vi "fit_fix height and width.vi"() -> ()   [LabVIEW 2016] (continued)
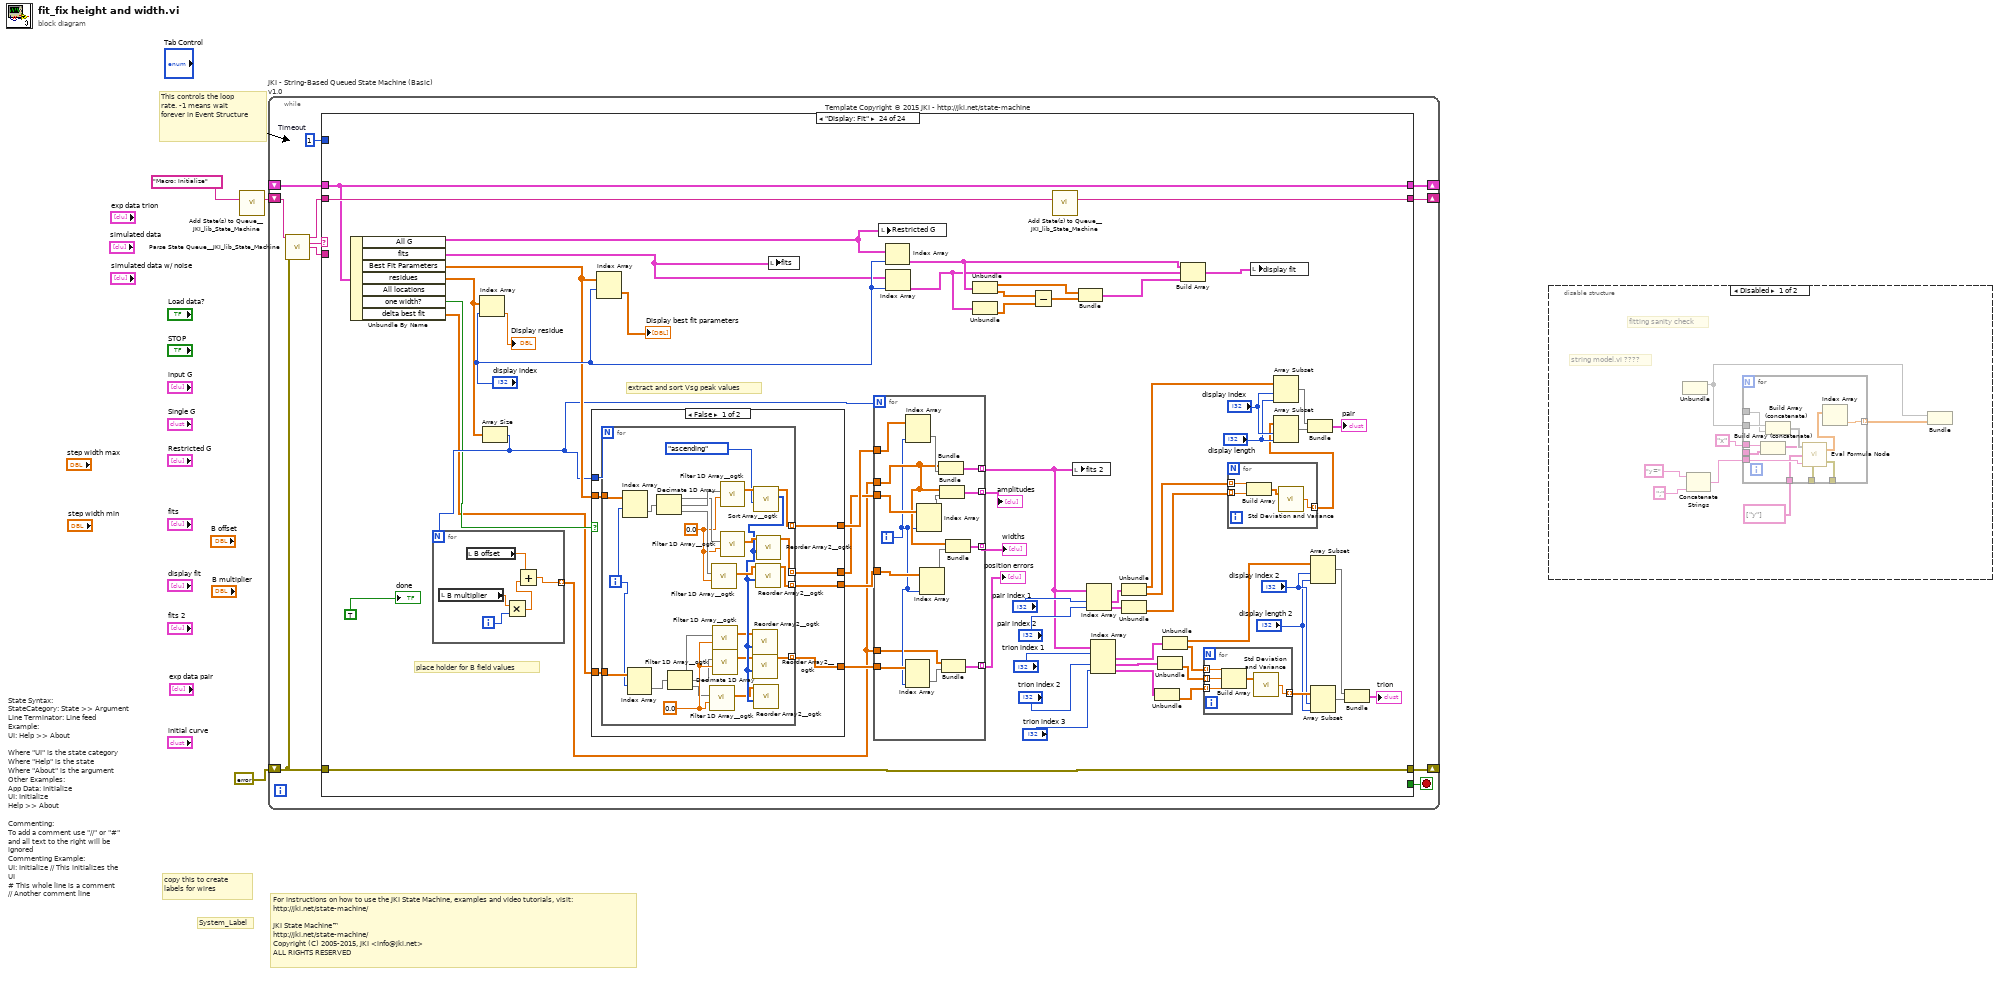
[diagram p0: block diagram]
diagram:
  # "For instructions on how to use the JKI State Machine, examples and video tutorials, visit:\nhttp://jki.net/state-machine/\n\nJKI State Machine™\nhttp://jki.net/state-machine/\nCopyright (C) 2005-2015, JKI <info@jki.net>\nALL RIGHTS RESERVED"
  # "State Syntax:\nStateCategory: State >> Argument\nLine Terminator: Line feed\nExample:\nUI: Help >> About\n\nWhere \"UI\" is the state category\nWhere \"Help\" is the state\nWhere \"About\" is the argument\nOther Examples:\nApp Data: Initialize\nUI: Initialize\nHelp >> About\n\nCommenting:\nTo add a comment use \"//\" or \"#\" and all text to the right will be ignored\nCommenting Example:\nUI: Initialize // This initializes the UI\n# This whole line is a comment\n// Another comment line"
  # "copy this to create labels for wires"
  # "This controls the loop rate. -1 means wait forever in Event Structure"
  # "System_Label"
  n1 = call <vilib>:"Add State(s) to Queue__JKI_lib_State_Machine.vi"("State(s) in (\"\")"="Macro: Initialize") -> ("States Out"=w3:string)  [unwired: 14 in]
  n2 = while "JKI - String-Based Queued State Machine (Basic) v1.0" {
    shift-right: [w7] -> _
    shift-left: _ -> [w6]
    shift-right: [w10] -> _
    shift-left: errorcluster {"status"=FALSE, "code"=0, "source"=""} ("error out") -> [w4]
    shift-right: [w9] -> _
    shift-left: w3 -> [w11]
    stop <- w8 stop-if-true
    w5 = 1  # Timeout
    # "Template Copyright © 2015 JKI - http://jki.net/state-machine"
    n3 = call <vilib>:"Parse State Queue__JKI_lib_State_Machine.vi"("State Queue"=w11, "Error In (no error)"=w4) -> ("Remaining States"=w13:string, "Current State"=w14:string, "Arguments"=w12:string)  [unwired: 11 in]
    n4 = case shown="\"Display: Fit\"" w14 {
      selector: w14 -> [_ _ w66 _ _ _ _ _ _ _ _ _ _ _ _ _ _ _ _ _ _ _ _ _]
      tunnel: w13 -> [w21 w65 w70 w88 w94 w100 w104 w135 w141 w145 w157 w163 w174 w200 w205 w215 w219 w248 w275 w312 w517 w593 w665 w726]
      tunnel: w12 -> [_ _ _ _ _ _ _ _ _ _ _ w158 w168 _ _ _ _ _ _ _ _ _ _ _]
      tunnel: w6 -> [w19 w62 w68 w79 w89 w98 w101 _ w136 w142 w154 w161 w170 w197 w202 w212 w216 w243 w271 w306 w511 w590 w662 w723]
      tunnel: [w18 w63 w72 w85 errorcluster {"status"=FALSE, "code"=0, "source"=""} ("error out") w97 w102 w132 w137 w143 w155 w159 w171 w198 w203 w213 w217 w246 w273 w310 w493 w589 w663 w720] -> w10
      tunnel: w4 -> [w17 w63 w71 w85 w90 w97 w102 w132 w138 w143 w155 w160 w172 w198 w203 w213 w217 w246 w273 w310 w510 w589 w663 w720]
      tunnel: [w20 w64 w69 w87 w93 w99 w103 w134 w140 w144 w156 w162 w173 w199 w204 w214 w218 w247 w274 w311 w516 w592 w664 w725] -> w9
      tunnel: [_ _ _ _ _ TRUE _ _ _ _ _ _ _ _ _ _ _ _ _ _ _ _ _ _] -> w8
      tunnel: [w16 w62 w68 w86 w89 w98 w101 w133 w136 w142 w152 w161 w170 w197 w202 w212 w216 w245 w270 w304 w514 w591 w662 w723] -> w7
      tunnel: w5 -> [w15 _ _ _ _ _ _ _ _ _ _ _ _ _ _ _ _ _ _ _ _ _ _ _]
      frame "", "Event Structure", "Idle" {
        # "executes when the state queue is empty"
        n5 = event shown="[0] Timeout" {
          selector: _ -> [_ _ _ _ _]
          dyn-events: _ -> [_ _ _ _ _]
          timeout: w15 -> [_ _ _ _ _]
          tunnel: w21 -> [w30 w35 w42 w55 w61]
          tunnel: [w29 w34 w41 w54 w60] -> w20
          tunnel: w19 -> [w24 w32 w38 w51 w58]
          tunnel: [w28 w33 w40 w53 w59] -> w18
          tunnel: w17 -> [w28 w33 w40 w53 w59]
          tunnel: [w22 w32 w39 w51 w58] -> w16
          event Timeout {
            n6 = event-data() -> ()  [unwired: 1 in, 1 out]
            n7 = local read "input G"() -> (w26:cluster{dbl[], dbl[]}[])
            n8 = Index Array(array=w26, index="choose initial curve") -> (element=w23:cluster{dbl[], dbl[]})
            n9 = Bundle By Name(cluster=w24, "initial curve"=w23) -> (w22:T5)
            n10 = local write "initial curve"(w23) -> ()
            n11 = call <vilib>:"Add State(s) to Queue__JKI_lib_State_Machine.vi"("State(s) in (\"\")"=w30, "State(s) at Back (\"\")"="Display: Fit" ("State(s) at Back (\"\")")) -> ("States Out"=w29:string)  [unwired: 13 in]
          }
          event "STOP": Value Change {
            # "Exit Button Value Change (pressed) Event\n(this executes Macro: Exit to terminate the VI)"
            n12 = event-data() -> ()  [unwired: 1 in, 1 out]
            n13 = call <vilib>:"Add State(s) to Queue__JKI_lib_State_Machine.vi"("State(s) in Front (\"\")"="Macro: Exit", "State(s) in (\"\")"=w35) -> ("States Out"=w34:string)  [unwired: 13 in]
          }
          event "Load data?": Value Change {
            n14 = event-data() -> ("NewVal"=w36:bool)  [unwired: 1 in, 5 out]
            n15 = case shown="True" w36 {
              tunnel: [w43 w50] -> w39
              tunnel: w38 -> [w43 w49]
              tunnel: [_ "UI: Initialize\nAnalysis: Load data"] -> w37
              frame False {
              }
              frame True {
                w47 = FALSE ("Done?")
                n16 = local write "done"(w47) -> ()
                n17 = Bundle By Name(cluster=w49, "curve #"=0, "Done?"=w47, "fits"=cluster{dbl[], dbl[]}[] [], "Initial curve?"=TRUE) -> (w50:T5)
              }
            }
            n18 = call <vilib>:"Add State(s) to Queue__JKI_lib_State_Machine.vi"("State(s) in Front (\"\")"=w37, "State(s) in (\"\")"=w42) -> ("States Out"=w41:string)  [unwired: 13 in]
          }
          event "display index": Value Change {
            n19 = event-data() -> ()  [unwired: 1 in, 6 out]
            n20 = call <vilib>:"Add State(s) to Queue__JKI_lib_State_Machine.vi"("State(s) in Front (\"\")"="Display: Fit", "State(s) in (\"\")"=w55) -> ("States Out"=w54:string)  [unwired: 13 in]
          }
          event Panel Close? {
            # "Discard the event because we'll close the front panel ourselves in Macro: Exit"
            # "Close Panel button (pressed) Event\n(this executes Macro: Exit to terminate the VI)"
            n21 = event-data() -> ()  [unwired: 1 in, 1 out]
            n22 = event-data("Discard?"=TRUE) -> ()  [unwired: 1 in, 1 out]
            n23 = call <vilib>:"Add State(s) to Queue__JKI_lib_State_Machine.vi"("State(s) in Front (\"\")"="Macro: Exit", "State(s) in (\"\")"=w61) -> ("States Out"=w60:string)  [unwired: 13 in]
          }
        }
      }
      frame "---------- Core ----------" {
        # "Do not put any code in this frame.\n(it is a separator no-op)"
        n24 = call <vilib>:"Add State(s) to Queue__JKI_lib_State_Machine.vi"("State(s) in (\"\")"=w65) -> ("States Out"=w64:string)  [unwired: 14 in]
      }
      frame Default {
        w75 = 42 items=["No error", "Argument error", "Memory is full", "Out of zone", "End of file", "File already open", "Generic file I/O error", "File not found", "File permission error", "Disk is full", "Duplicate path", "Too many files open", "System feature not enabled", "Resource file not found", "Cannot add resource", "Resource not found", "Image not found", "Image memory error", "Pen does not exist", "Config type invalid", "Config token not found", "Config parse error", "Config memory error", "Bad external code format", "Bad external code offset", "External code not present", "Null window", "Destroy window error", "Null menu", "Print aborted", "Bad print record", "Print driver error", "Windows error during printing", "Memory error during printing", "Print dialog error", "Generic print error", "Invalid device refnum", "Device not found", "Device parameter error", "Device unit error", "Cannot open device", "Device call aborted", "Generic error", "Cancelled by user", "Object ID too low", "Object ID too high", "Object not in heap", "Unknown heap", "Unknown object (invalid DefProc)", "Unknown object (DefProc not in table)", "Message out of range", "Invalid (null) method", "Unknown message", "Manager call not supported", "Bad address", "Network operation in progress", "Network operation timed out", "Connection is busy", "Network attribute not supported", "Network error", "Address in use", "System out of memory", "Connection aborted", "Connection refused", "Not connected", "Already connected", "Connection closed", "Initialization error (interapplication manager)", "Bad occurrence", "Wait on unbound occurrence handler", "Occurrence queue overflow", "Datalog type conflict", "Unused", "Unrecognized type (interapplication manager)", "Memory corrupt", "Failed to make temporary DLL", "Old CIN version", "Drag socket not found", "Failed to load drop-object", "Failed to register OLE object", "Failed to release OLE object", "Format specifier type mismatch", "Unknown format specifier", "Too few format specifiers", "Too many format specifiers", "Scan failed", "Newer CIN version", "Error converting to variant", "Runtime menu error", "Password tampered", "Variant attribute not found", "Incompatible variant data type", "Event data is not available", "Event Store is not present", "Occurrence is not found", "Event Queue is not created", "Event info is not available", "Refnum passed is NULL", "Error retrieving Class GUID", "Error retrieving CoClass GUID", "Error retrieving TypeLib GUID.", "Bad built application magic bytes.", "Specific driver is different from the specific driver associated with the Logical Name.", "There is no session opened to the class driver.", "Max Error", "MAX - Error with config objects", "MAX - Error loading configuration", "MAX - Group not supported"]
        # "Current State"
        # "Do not delete, rename, or modify this frame.\n(this is used to capture unhandled states and typos)"
        # "Handle mistyped state name (developer tool)"
        n25 = Format Into String(format string="Software Exception: Unhandled State \"%s\"." ("message"), error in=w71, w66) -> (resulting string=w74:string, error out=w73:errorcluster)  [unwired: 1 in]
        n26 = call <vilib>:"Error Cluster From Error Code.vi"("show call chain? (False)"=TRUE, "error in (no error)"=w73, "error message (\"\")"=w74, "error code (0)"=w75) -> ("error out"=w72:errorcluster)  [unwired: 5 in]
        n27 = call <vilib>:"Add State(s) to Queue__JKI_lib_State_Machine.vi"("State(s) in (\"\")"=w70) -> ("States Out"=w69:string)  [unwired: 14 in]
      }
      frame "Initialize Core Data" {
        # "Do not delete, rename, or modify this frame.\n(this is used to determine panel behavior on exit)"
        # "originally closed?"
        # "exe?"
        # "If panel starts closed or is an EXE, then close it when we exit"
        n28 = property class="App"() -> ("App.Kind"=w83:T3)  [unwired: 2 in, 2 out]
        n29 = property class="VI"() -> ("Front Panel.Open"=w84:bool)  [unwired: 2 in, 2 out]
        n30 = control-ref of="Current VI Reference"() -> (w77:refnum<vi>)
        n31 = Not(x=w84) -> (.not. x?=w81:bool)
        n32 = Equal?(x=w83, y=T3."Run Time System" ("Application:Kind")) -> (x = y?=w80:bool)
        n33 = Or(x=w81, y=w80) -> (x .or. y?=w78:bool)
        n34 = Bundle By Name(cluster=w79, "Core.Current VI Reference"=w77, "Core.Close Panel on Exit?"=w78) -> (w86:T5)
        n35 = call <vilib>:"Add State(s) to Queue__JKI_lib_State_Machine.vi"("State(s) in (\"\")"=w88) -> ("States Out"=w87:string)  [unwired: 14 in]
      }
      frame "Error Handler" {
        # "Unhandled Error -- Display it"
        # "Handle any errors here.\nYou can also output any states to clean-up after errors occur"
        # "Clear error"
        n36 = disable-structure shown="Disabled" {
          disable-tunnel: w90 -> [w95 _]
          frame Disabled {
            n37 = call <vilib>:"General Error Handler.vi"("error in (no error)"=w95) -> ()  [unwired: 10 in, 5 out]
          }
          frame Enabled {
          }
        }
        n38 = call <vilib>:"Add State(s) to Queue__JKI_lib_State_Machine.vi"("State(s) in (\"\")"=w94, "State(s) at Back (\"\")"="/* Post Error States") -> ("States Out"=w93:string)  [unwired: 13 in]
      }
      frame "Exit" {
        # "Do not put any code in this frame.\n(No errors that occur here will be handled.)"
        n39 = call <vilib>:"Add State(s) to Queue__JKI_lib_State_Machine.vi"("State(s) in (\"\")"=w100) -> ("States Out"=w99:string)  [unwired: 14 in]
      }
      frame "---------- Data ----------" {
        # "Do not put any code in this frame.\n(It is a separator no-op. You can make a copy of this frame to create a new Data frame)"
        n40 = call <vilib>:"Add State(s) to Queue__JKI_lib_State_Machine.vi"("State(s) in (\"\")"=w104) -> ("States Out"=w103:string)  [unwired: 14 in]
      }
      frame "Data: Initialize" {
        w105 = dbl[][] []  # delta best fit
        w106 = dbl[][] []  # Intermediate delta
        w107 = FALSE  # one width?
        w108 = i32[] []  # Fit steps
        w109 = dbl[][] []  # All locations
        w110 = dbl[] []  # Initial Best Fit
        w111 = FALSE  # Initial curve?
        w112 = cluster{"Single G curve":dbl[], dbl[]} {"Single G curve"=[], []}  # initial curve
        w114 = dbl[] []  # intermediate residues
        w115 = cluster{dbl[], dbl[]}[] []  # intermediate fits
        w116 = dbl[][] []  # Intermediate Best Fit
        w118 = 0  # fit iteration
        w119 = dbl[] []  # residues
        w120 = cluster{"max iteration":i32, "tolerance":dbl} {"max iteration"=200, "tolerance"=1e-08}  # termination
        w121 = T6 {"parameter minimum"=[], "parameter maximum"=[]}  # parameter bounds
        w122 = 0  # model step #
        w123 = dbl[][] []  # Best Fit Parameters
        w124 = dbl[] []  # Initial Parameters
        w125 = dbl[] []  # Locations
        w126 = dbl[] []  # Locations index
        w117 = -1  # curve #
        w127 = cluster{"Single G curve":dbl[], dbl[]} {"Single G curve"=[], []}  # Single G curve
        w128 = cluster{dbl[], dbl[]}[] []  # All G
        w129 = T7 {"Current VI Reference"=refnum, "Close Panel on Exit?"=FALSE}  # Core
        w131 = TRUE  # Done?
        w130 = ""  # Your string data
        # "Initialize the shift-register data, here.\n(data names are defined by what you wire into the bundle function)"
        n41 = local read "fits"() -> (w113:cluster{dbl[], dbl[]}[])
        n42 = call <vilib>:"Add State(s) to Queue__JKI_lib_State_Machine.vi"("State(s) in (\"\")"=w135) -> ("States Out"=w134:string)  [unwired: 14 in]
        n43 = Bundle("Core"=w129, "Done?"=w131, "Your string data"=w130, "All G"=w128, "Single G curve"=w127, "Locations index"=w126, "Locations"=w125, "Initial Parameters"=w124, "Best Fit Parameters"=w123, "Intermediate Best Fit"=w116, "curve #"=w117, "fits"=w113, "intermediate fits"=w115, "model step #"=w122, "parameter bounds"=w121, "termination"=w120, "residues"=w119, "intermediate residues"=w114, "fit iteration"=w118, "initial curve"=w112, "Initial curve?"=w111, "Initial Best Fit"=w110, "All locations"=w109, "Fit steps"=w108, "one width?"=w107, "delta best fit"=w105, "Intermediate delta"=w106) -> (w133:T5)  [unwired: 1 in]
      }
      frame "Data: Cleanup" {
        # "Cleanup any data and references, here.\n(this is called automatically, by the Macro: Exit)"
        n44 = Unbundle By Name(w136) -> ("Core.Current VI Reference"=w139:refnum<vi>)
        n45 = Close Reference(reference=w139, error in (no error)=w138) -> (error out=w137:errorcluster)
        n46 = call <vilib>:"Add State(s) to Queue__JKI_lib_State_Machine.vi"("State(s) in (\"\")"=w141) -> ("States Out"=w140:string)  [unwired: 14 in]
      }
      frame "---------- UI ----------" {
        # "Do not put any code in this frame.\n(It is a separator no-op. You can make a copy of this frame to create a new UI frame)"
        n47 = call <vilib>:"Add State(s) to Queue__JKI_lib_State_Machine.vi"("State(s) in (\"\")"=w145) -> ("States Out"=w144:string)  [unwired: 14 in]
      }
      frame "UI: Initialize" {
        # "default termination conditions"
        # "Initialize the User Interface, here.\n(this is called automatically, by the Macro: Init)"
        n48 = Bundle By Name(cluster=w154, "intermediate fits"=cluster{dbl[], dbl[]}[] [] ("fits"), "Best Fit Parameters"=dbl[][] [], "Intermediate Best Fit"=dbl[][] [] ("Best Fit Parameters"), "residues"=dbl[] [], "fit iteration"=0, "termination"=cluster{"max iteration":i32, "tolerance":dbl} {"max iteration"=200, "tolerance"=1e-08}, "Fit steps"=i32[] []) -> (w152:T5)
        n49 = call <vilib>:"Add State(s) to Queue__JKI_lib_State_Machine.vi"("State(s) in (\"\")"=w157) -> ("States Out"=w156:string)  [unwired: 14 in]
      }
      frame "UI: Cursor Set" {
        # "Argument"
        # "Set and Unset Cursor Busy.\n(Usage: \"UI: Cursor Set >> Busy|Idle\")"
        n50 = case shown="\"Idle\", Default" w158 {
          tunnel: w160 -> [w165 w167]
          tunnel: [w164 w166] -> w159
          frame "Idle", Default {
            n51 = call <vilib>:"Unset Busy.vi"("error in (no error)"=w165) -> ("error out"=w164:errorcluster)  [unwired: 10 in]
          }
          frame "Busy" {
            n52 = call <vilib>:"Set Busy.vi"("error in (no error)"=w167) -> ("error out"=w166:errorcluster)  [unwired: 9 in, 1 out]
          }
        }
        n53 = call <vilib>:"Add State(s) to Queue__JKI_lib_State_Machine.vi"("State(s) in (\"\")"=w163) -> ("States Out"=w162:string)  [unwired: 14 in]
      }
      frame "UI: Front Panel State" {
        # "Argument"
        # "Set Front Panel Open or Closed\n(Usage: \"UI: Front Panel State >> Open|Close\")"
        n54 = Unbundle By Name(w170) -> ("Core.Current VI Reference"=w169:refnum<vi>)
        n55 = case shown="\"Open\", Default" w168 {
          tunnel: w172 -> [w178 w191]
          tunnel: [w180 w192] -> w171
          tunnel: w169 -> [w179 w189]
          frame "Open", Default {
            n56 = property class="VI"(reference=w179, error in=w178) -> (reference out=w176:refnum<vi>, error out=w177:errorcluster, "Front Panel.Open"=w175:bool)
            n57 = case shown="False" w175 {
              tunnel: [w183 w186] -> w180
              tunnel: w177 -> [w182 w186]
              tunnel: w176 -> [w181 _]
              frame False {
                n58 = invoke class="VI" method="FP.Open"(reference=w181, error in=w182, "Activate"=TRUE, "State"=T4."Standard") -> (error out=w183:errorcluster)  [unwired: 1 in, 4 out]
              }
              frame True {
              }
            }
          }
          frame "Close" {
            n59 = property class="VI"(reference=w189, error in=w191) -> (reference out=w188:refnum<vi>, error out=w190:errorcluster, "Front Panel.Open"=w187:bool)
            n60 = case shown="True" w187 {
              tunnel: [w193 w196] -> w192
              tunnel: w190 -> [w193 w195]
              tunnel: w188 -> [_ w194]
              frame False {
              }
              frame True {
                n61 = invoke class="VI" method="FP.Close"(reference=w194, error in=w195) -> (error out=w196:errorcluster)  [unwired: 1 in, 2 out]
              }
            }
          }
        }
        n62 = call <vilib>:"Add State(s) to Queue__JKI_lib_State_Machine.vi"("State(s) in (\"\")"=w174) -> ("States Out"=w173:string)  [unwired: 14 in]
      }
      frame "---------- Macro ----------" {
        # "Do not put any code in this frame.\n(It is a separator no-op. You can make a copy of this frame to create a new Macro frame)"
        n63 = call <vilib>:"Add State(s) to Queue__JKI_lib_State_Machine.vi"("State(s) in (\"\")"=w200) -> ("States Out"=w199:string)  [unwired: 14 in]
      }
      frame "Macro: Initialize" {
        w201 = "Data: Initialize\nInitialize Core Data\nUI: Initialize\nUI: Front Panel State >> Open"  # Data: Initialize Initialize Core Data UI: Initialize UI: Front Panel State >> Open
        # "Initialization Macro\n(This is called once, when the VI starts)"
        n64 = call <vilib>:"Add State(s) to Queue__JKI_lib_State_Machine.vi"("State(s) in Front (\"\")"=w201, "State(s) in (\"\")"=w205) -> ("States Out"=w204:string)  [unwired: 13 in]
      }
      frame "Macro: Exit" {
        # "Exit Macro\n(This is called once, when the VI exits)"
        n65 = Unbundle By Name(w212) -> ("Core.Close Panel on Exit?"=w211:bool)
        n66 = Select(t="UI: Front Panel State >> Close", s=w211, f="") -> (s? t:f=w208:string)
        n67 = call <vilib>:"Add State(s) to Queue__JKI_lib_State_Machine.vi"("State(s) in (\"\")"=w208, "State(s) at Back (\"\")"="Data: Cleanup\nExit") -> ("States Out"=w206:string)  [unwired: 13 in]
        n68 = call <vilib>:"Add State(s) to Queue__JKI_lib_State_Machine.vi"("State(s) in Front (\"\")"=w206, "State(s) in (\"\")"=w215) -> ("States Out"=w214:string)  [unwired: 13 in]
      }
      frame "---------- Analysis ----------" {
        # "Template Separator\n(You can make a copy of, or modify, this frame)"
        n69 = call <vilib>:"Add State(s) to Queue__JKI_lib_State_Machine.vi"("State(s) in (\"\")"=w219) -> ("States Out"=w218:string)  [unwired: 14 in]
      }
      frame "Analysis: Load data" {
        # "Load data and step through curves for fitting"
        n70 = local read "input G"() -> (w230:cluster{dbl[], dbl[]}[])
        n71 = Unbundle By Name(w243) -> ("curve #"=w229:i32, "fit iteration"=w225:i32, "Initial curve?"=w233:bool)
        "curve #" <- w229
        n72 = Array Size(array=w230) -> (size(s)=w228:i32)
        n73 = Decrement(x=w228) -> (x-1=w227:i32)
        n74 = case shown="True" "Restrict G?" {
          tunnel: w230 -> [w249 w251]
          tunnel: [w249 w250] -> w242
          frame False {
          }
          frame True {
            n75 = for {
              tunnel: w251 -> [w259] mode=indexing
              tunnel: [w252] -> w250 mode=indexing
              n76 = Unbundle(w259) -> (w257:dbl[], w256:dbl[])
              n77 = Threshold 1D Array(2:"Max G", 3:w256) -> (0:w255:dbl)  [unwired: 1 in]
              n78 = Array Subset(array=w256, length=w255) -> (w253:dbl[])  [unwired: 1 in]
              n79 = Array Subset(array=w257, length=w255) -> (w254:dbl[])  [unwired: 1 in]
              n80 = Bundle(w254, w253) -> (w252:cluster{dbl[], dbl[]})  [unwired: 1 in]
            }
          }
        }
        n81 = Equal?(x=w229, y=w227) -> (x = y?=w226:bool)
        n82 = Equal?(x=w225, y=0) -> (x = y?=w223:bool)
        n83 = And(x=w226, y=w223) -> (x .and. y?=w222:bool)
        n84 = local read "choose initial curve"() -> (w232:i32)
        n85 = case shown="True" w222 {
          frame False {
          }
          frame True {
            n86 = call <vilib>:"Beep.vi"() -> ()  [unwired: 12 in]
          }
        }
        n87 = Select(t=w232, s=w233, f=w229) -> (s? t:f=w231:i32)
        n88 = Index Array(array=w242, index=w231) -> (element=w234:cluster{dbl[], dbl[]})
        n89 = local write "Single G"(w234) -> ()
        n90 = local write "Restricted G"(w242) -> ()
        n91 = Unbundle(w234) -> (w240:dbl[])  [unwired: 1 out]
        n92 = Array Max & Min(array=w240) -> (max value=w241:dbl)  [unwired: 3 out]
        n93 = Round Toward -Infinity(1:w241) -> (0:w221:dbl)
        n94 = Add(x=w221, y=w225) -> (x+y=w239:dbl)
        n95 = Bundle By Name(cluster=w243, "All G"=w242, "Single G curve"=w234, "model step #"=w239) -> (w245:T5)
        n96 = Equal?(x=0, y=w225) -> (x = y?=w237:bool)
        n97 = Select(t="Analysis: find peaks" ("State(s) at Back (\"\")"), s=w237, f="Analysis: Initial Parameters" ("State(s) at Back (\"\")")) -> (s? t:f=w220:string)
        n98 = call <vilib>:"Add State(s) to Queue__JKI_lib_State_Machine.vi"("State(s) in Front (\"\")"=w220, "State(s) in (\"\")"=w248) -> ("States Out"=w247:string)  [unwired: 13 in]
      }
      frame "Analysis: find peaks" {
        # "Fid peak locations to help constrain step position inital parameters"
        n99 = Unbundle By Name(w271) -> ("Single G curve"=w272:cluster{"Single G curve":dbl[], dbl[]})
        n100 = call <userlib>:"differential.vi"("Numeric"="derivative \nfor peak initial conditions", "dy/dx vs x"=TRUE, "A vs B 2"=w272) -> ("A vs B 3"=w267:T8)  [unwired: 1 in]
        n101 = Unbundle(w267) -> ("Decimated Array"=w263:dbl[], "Decimated Array"=w266:dbl[])
        n102 = call <vilib>:"Peak Detector.vi"("width"="derivative peak width", "threshold"="derivative peak threshold", "X"=w266) -> ("Locations"=w262:dbl[])  [unwired: 4 in, 4 out]
        "Locations index" <- w262
        n103 = for {
          N -> [w276]
          tunnel: w263 -> [w279]
          tunnel: w262 -> [w278] mode=indexing
          tunnel: [w277] -> w261 mode=indexing
          tunnel: [w276] -> _ mode=indexing
          n104 = Interpolate 1D Array(1:w278, 2:w279) -> (0:w277:dbl)
        }
        "Locations" <- w261
        n105 = call <vilib>:"Add State(s) to Queue__JKI_lib_State_Machine.vi"("State(s) in Front (\"\")"="Analysis: Initial Parameters" ("State(s) at Back (\"\")"), "State(s) in (\"\")"=w275) -> ("States Out"=w274:string)  [unwired: 13 in]
        n106 = Bundle By Name(cluster=w271, "Locations index"=w262, "Locations"=w261) -> (w270:T5)
      }
      frame "Analysis: Initial Parameters" {
        # "Create initial parameter and parameter bound arrays"
        n107 = Unbundle By Name(w306) -> ("Initial Best Fit"=w297:dbl[], "Initial curve?"=w288:bool, "model step #"=w301:i32, "Single G curve"=w309:cluster{"Single G curve":dbl[], dbl[]}, "Locations index"=w308:dbl[], "Locations"=w307:dbl[], "Best Fit Parameters"=w292:dbl[][], "residues"=w291:dbl[], "curve #"=w281:i32)
        n108 = case shown="True" "fix step width?" {
          tunnel: [w315 w316] -> w296
          tunnel: [w314 w316] -> w295
          tunnel: ["step width?" w316] -> w284
          tunnel: w281 -> [_ w324]
          frame False {
            n109 = local read "step width max"() -> (w315:dbl)
            n110 = local read "step width min"() -> (w314:dbl)
          }
          frame True {
            n111 = local read "B multiplier"() -> (w323:dbl)
            n112 = local read "B offset"() -> (w321:dbl)
            n113 = Multiply(x=w324, y=w323) -> (x*y=w322:dbl)
            n114 = Add(x=w322, y=w321) -> (x+y=w319:dbl)
            n115 = Multiply(x=w319, y="fix width slope") -> (x*y=w317:dbl)
            n116 = Add(x=w317, y="fix width intercept") -> (x+y=w316:dbl)
          }
        }
        n117 = Array Size(array=w291) -> (size(s)=w290:i32)
        n118 = Unbundle(w309) -> ("Single G curve"=w302:dbl[], w303:dbl[])
        n119 = Select(t=w288, s="fit inital parameters?", f=TRUE) -> (s? t:f=w287:bool)
        n120 = Decrement(x=w290) -> (x-1=w289:i32)
        n121 = case shown="True" w287 {
          tunnel: w308 -> [w339 w400]
          tunnel: w307 -> [w338 w399]
          tunnel: [w347 w398] -> w305
          tunnel: w303 -> [w341 w397]
          tunnel: w302 -> [w344 w396]
          tunnel: w301 -> [w351 w395]
          tunnel: [w337 w394] -> w300
          tunnel: [w345 w393] -> w299
          tunnel: w297 -> [w348 _]
          tunnel: w296 -> [w336 w392]
          tunnel: w295 -> [w335 w391]
          tunnel: "step height max" -> [w334 w390]
          tunnel: "step height min" -> [w333 w389]
          tunnel: w292 -> [w332 _]
          tunnel: w289 -> [w331 _]
          tunnel: "one width?" -> [_ w388]
          tunnel: w284 -> [_ w387]
          frame False {
            w346 = dbl[] []
            n122 = Index Array(array=w332, index (row)=w331) -> (element=w330:dbl[])  [unwired: 1 in]
            n123 = Array Max & Min(array=w344) -> (max value=w343:dbl, min value=w342:dbl)  [unwired: 2 out]
            n124 = call-poly <userlib>:"Filter 1D Array__ogtk.vi"("items to filter"=0.0, "array"=w348) -> ("filtered array"=w352:dbl[])  [unwired: 4 in, 1 out]
            n125 = Decimate 1D Array(w330) -> (w328:dbl[])  [unwired: 2 out]
            n126 = Multiply(x=w328, y="Max position %") -> (x*y=w326:dbl[])
            n127 = Multiply(x=w328, y="Min position %") -> (x*y=w325:dbl[])
            n128 = Decimate 1D Array(w352) -> (w350:dbl[], w349:dbl[])  [unwired: 1 out]
            n129 = for {
              N: w351 -> [_]
              tunnel: w350 -> [w386]
              tunnel: w349 -> [w385]
              shift-right: [w383] -> w347
              shift-left: dbl[] [] -> [w384]
              shift-right: [w381] -> w345
              shift-left: w346 -> [w382]
              shift-right: [w379] -> w337
              shift-left: w346 -> [w380]
              tunnel: w343 -> [w371]
              tunnel: w342 -> [w368]
              tunnel: w341 -> [w378]
              tunnel: w339 -> [w377]
              tunnel: w338 -> [w375]
              tunnel: w336 -> [w360]
              tunnel: w335 -> [w359]
              tunnel: w334 -> [w362]
              tunnel: w333 -> [w361]
              tunnel: w326 -> [w367]
              tunnel: w325 -> [w365]
              i -> [w364]
              n130 = Index Array(array=w367, index=w364) -> (element=w366:dbl)
              n131 = Index Array(array=w365, index=w364) -> (element=w363:dbl)
              n132 = Index Array(array=w386, index=w364) -> (element=w356:dbl)
              n133 = Index Array(array=w385, index=w364) -> (element=w372:dbl)
              n134 = Threshold 1D Array(2:w364, 3:w378) -> (0:w376:dbl)  [unwired: 1 in]
              n135 = call "compare if zero.vi"("if zero out"=w368, "Numeric"=w363) -> ("out"=w369:dbl)  [unwired: 5 in]
              n136 = call "compare if zero.vi"("if zero out"=w362, "Numeric"=w356) -> ("out"=w358:dbl)  [unwired: 5 in]
              n137 = call "compare if zero.vi"("if zero out"=w371, "Numeric"=w366) -> ("out"=w370:dbl)  [unwired: 5 in]
              n138 = call "Search 1D Array for Nearest LV2012 NIVerified.vi"("desired element"=w376, "1D Array"=w377) -> ("closest index"=w374:i32)  [unwired: 8 in, 1 out]
              n139 = call "compare if zero.vi"("if zero out"=w360, "Numeric"=w372) -> ("out"=w355:dbl)  [unwired: 5 in]
              n140 = call "compare if zero.vi"("if zero out"=w361, "Numeric"=w356) -> ("out"=w357:dbl)  [unwired: 5 in]
              n141 = call "compare if zero.vi"("if zero out"=w359, "Numeric"=w372) -> ("out"=w354:dbl)  [unwired: 5 in]
              n142 = Index Array(array=w375, index=w374) -> (element=w373:dbl)
              n143 = Build Array (concatenate)(w382, w358, w370, w355) -> (w381:dbl[])
              n144 = Build Array (concatenate)(w380, w357, w369, w354) -> (w379:dbl[])
              n145 = Build Array (concatenate)(w384, w356, w373, w372) -> (w383:dbl[])
            }
          }
          frame True {
            n146 = case shown="True" w388 {
              tunnel: w400 -> [w418 w453]
              tunnel: w399 -> [w417 w452]
              tunnel: [w416 w451] -> w398
              tunnel: w397 -> [w415 w450]
              tunnel: w396 -> [w414 w448]
              tunnel: w395 -> [w411 w445]
              tunnel: [w410 w444] -> w394
              tunnel: [w409 w443] -> w393
              tunnel: w392 -> [w404 w441]
              tunnel: w391 -> [w402 w440]
              tunnel: w390 -> [w408 w439]
              tunnel: w389 -> [w407 w438]
              tunnel: w387 -> [w406 w437]
              frame True {
                n147 = Array Max & Min(array=w414) -> (max value=w413:dbl, min value=w412:dbl)  [unwired: 2 out]
                n148 = Build Array(w406) -> (w405:dbl[])
                n149 = Build Array(w404) -> (w403:dbl[])
                n150 = Build Array(w402) -> (w401:dbl[])
                n151 = for {
                  N: w411 -> [_]
                  tunnel: w415 -> [w436]
                  shift-right: [w428] -> w416
                  shift-left: w405 -> [w429]
                  tunnel: w418 -> [w434]
                  tunnel: w417 -> [w432]
                  shift-right: [w426] -> w409
                  shift-left: w403 -> [w427]
                  shift-right: [w425] -> w410
                  shift-left: w401 -> [w424]
                  tunnel: w413 -> [w423]
                  tunnel: w412 -> [w421]
                  tunnel: w404 -> [_]
                  tunnel: w402 -> [_]
                  tunnel: w408 -> [w420]
                  tunnel: w407 -> [w419]
                  i -> [w435]
                  n152 = Threshold 1D Array(2:w435, 3:w436) -> (0:w433:dbl)  [unwired: 1 in]
                  n153 = call "Search 1D Array for Nearest LV2012 NIVerified.vi"("desired element"=w433, "1D Array"=w434) -> ("closest index"=w422:i32)  [unwired: 8 in, 1 out]
                  n154 = Index Array(array=w432, index=w422) -> (element=w430:dbl)
                  n155 = Build Array (concatenate)(w429, 1.0 ("element"), w430) -> (w428:dbl[])
                  n156 = Build Array (concatenate)(w427, w420, w423) -> (w426:dbl[])
                  n157 = Build Array (concatenate)(w424, w419, w421) -> (w425:dbl[])
                }
              }
              frame False {
                w442 = dbl[] []
                n158 = Array Max & Min(array=w448) -> (max value=w447:dbl, min value=w446:dbl)  [unwired: 2 out]
                n159 = for {
                  N: w445 -> [_]
                  tunnel: w450 -> [w474]
                  shift-right: [w466] -> w451
                  shift-left: dbl[] [] -> [w467]
                  tunnel: w453 -> [w472]
                  tunnel: w452 -> [w470]
                  shift-right: [w464] -> w443
                  shift-left: w442 -> [w465]
                  shift-right: [w463] -> w444
                  shift-left: w442 -> [w462]
                  tunnel: w447 -> [w461]
                  tunnel: w446 -> [w459]
                  tunnel: w441 -> [w458]
                  tunnel: w440 -> [w457]
                  tunnel: w439 -> [w456]
                  tunnel: w438 -> [w455]
                  tunnel: w437 -> [w454]
                  i -> [w473]
                  n160 = Threshold 1D Array(2:w473, 3:w474) -> (0:w471:dbl)  [unwired: 1 in]
                  n161 = call "Search 1D Array for Nearest LV2012 NIVerified.vi"("desired element"=w471, "1D Array"=w472) -> ("closest index"=w460:i32)  [unwired: 8 in, 1 out]
                  n162 = Index Array(array=w470, index=w460) -> (element=w468:dbl)
                  n163 = Build Array (concatenate)(w467, 1.0 ("element"), w468, w454) -> (w466:dbl[])
                  n164 = Build Array (concatenate)(w465, w456, w461, w458) -> (w464:dbl[])
                  n165 = Build Array (concatenate)(w462, w455, w459, w457) -> (w463:dbl[])
                }
              }
            }
          }
        }
        "Initial Parameters" <- w305
        n166 = Bundle(w300, w299) -> (w298:cluster{dbl[], dbl[]})  [unwired: 1 in]
        n167 = call <vilib>:"Add State(s) to Queue__JKI_lib_State_Machine.vi"("State(s) in Front (\"\")"="Analysis: Fit" ("State(s) at Back (\"\")"), "State(s) in (\"\")"=w312) -> ("States Out"=w311:string)  [unwired: 13 in]
        n168 = Bundle By Name(cluster=w306, "Initial Parameters"=w305, "parameter bounds"=w298, "one width?"="one width?") -> (w304:T5)
      }
      frame "Analysis: Fit" {
        (unwired) errorcluster {"status"=FALSE, "code"=0, "source"=""} ("error out")
        # "increase termination conditions \nif there is a max iteration error"
        # "Fit data"
        n169 = Unbundle By Name(w511) -> ("termination"=w498:cluster{"max iteration":i32, "tolerance":dbl}, "intermediate fits"=w501:cluster{dbl[], dbl[]}[], "Single G curve"=w508:cluster{"Single G curve":dbl[], dbl[]}, "Initial Parameters"=w515:dbl[], "Intermediate Best Fit"=w509:dbl[][], "intermediate residues"=w504:dbl[], "termination"=w506:cluster{"max iteration":i32, "tolerance":dbl}, "parameter bounds"=w507:T6, "Intermediate delta"=w484:dbl[][])
        "termination" <- w506
        n170 = case shown="\"normal tanh\", Default" "fit vi path" {
          tunnel: [path "C:/user/megan/hg/levylab_user_megan/data analysis/pascal fitting/subVI/LM model function and gradient_step.vi" ("vi path") path "C:/user/megan/hg/levylab_user_megan/data analysis/pascal fitting/subVI/LM model function_1 width.vi" ("vi path")] -> w485
          frame "normal tanh", Default {
          }
          frame "tanh w/ 1 width" {
          }
        }
        n171 = Unbundle(w508) -> ("Single G curve"=w481:dbl[], w482:dbl[])
        n172 = Open VI Reference(type specifier VI Refnum (for type only)=refnum<vi> refnum, vi path=w485) -> (vi reference=w512:refnum<vi>)  [unwired: 4 in, 1 out]
        n173 = call-by-ref "?"(reference=w512, "X"=w481, "a"=w515) -> (reference out=w479:refnum<vi>)  [unwired: 3 in, 4 out]
        n174 = Unbundle(w498) -> ("max iteration"=w497:i32, "tolerance"=w496:dbl)
        n175 = call-poly <vilib>:"Constrained Nonlinear Curve Fit.vi"("Y"=w482, "f(x,a)"=w479, "X"=w481, "initial parameters"=w515, "error in (no error)"=w510, "termination"=w506, "parameter bounds"=w507, "method"="method") -> ("best nonlinear fit"=w491:dbl[], "best fit parameters"=w480:dbl[], "residue"=w487:dbl, "error out"=w477:errorcluster)  [unwired: 2 in, 2 out]
        n176 = call <vilib>:"Goodness of Fit.vi"("Best Fit"=w491, "Y"=w482) -> ("RMSE"=→"RMSE":dbl, "R-square"=→"R-square":dbl, "SSE"=→"SSE":dbl)  [unwired: 6 in, 1 out]
        n177 = disable-structure shown="Disabled" {
          disable-tunnel: w482 -> [w523 _]
          disable-tunnel: w481 -> [w522 _]
          disable-tunnel: w480 -> [w521 _]
          disable-tunnel: w479 -> [w520 _]
          disable-tunnel: [w519 _] -> w478
          disable-tunnel: w477 -> [w518 _]
          frame Disabled {
            n178 = call <vilib>:"Nonlinear Curve Fit Intervals.vi"("Y"=w523, "f(x,a)"=w520, "X"=w522, "best fit parameters"=w521, "error in (no error)"=w518) -> ("delta best fit parameters"=w519:dbl[])  [unwired: 7 in, 3 out]
          }
          frame Enabled {
          }
        }
        n179 = Bundle("Single G curve"=w481, "best nonlinear fit"=w491) -> (w502:T9)  [unwired: 1 in]
        n180 = Equal?(x=errorcluster {"status"=TRUE, "code"=-23026, "source"="maximum iterations exceeded"} ("error out"), y=w477) -> (x = y?=w499:bool)
        n181 = case shown="True" w499 {
          tunnel: w509 -> [w541 w553]
          tunnel: w480 -> [w540 _]
          tunnel: [w539 w553] -> w505
          tunnel: w504 -> [w538 w552]
          tunnel: w487 -> [w537 _]
          tunnel: [w536 w552] -> w503
          tunnel: w502 -> [w535 _]
          tunnel: [w534 w551] -> w500
          tunnel: w501 -> [w533 w551]
          tunnel: w497 -> [w532 w547]
          tunnel: w496 -> [w531 w548]
          tunnel: [w531 w546] -> w494
          tunnel: [w532 w545] -> w495
          tunnel: ["Analysis: Iterate" "Analysis: Fit"] -> w475
          tunnel: w477 -> [w527 _]
          tunnel: [w527 errorcluster {"status"=FALSE, "code"=0, "source"=""} ("error out")] -> w493
          tunnel: w484 -> [w529 w542]
          tunnel: [w528 w542] -> w483
          tunnel: w480 -> [_ _]
          tunnel: w481 -> [_ _]
          tunnel: w482 -> [_ _]
          tunnel: w479 -> [_ _]
          tunnel: w478 -> [w526 _]
          frame False {
            n182 = Build Array (concatenate)(w541, w540) -> (w539:dbl[][])
            n183 = Build Array (concatenate)(w538, w537) -> (w536:dbl[])
            n184 = Build Array (concatenate)(w529, w526) -> (w528:dbl[][])
            n185 = Insert Into Array(array=w533, new element=w535) -> (w534:cluster{dbl[], dbl[]}[])  [unwired: 1 in]
          }
          frame True {
            n186 = Multiply(x=w548, y=2.0) -> (x*y=w546:dbl)
            n187 = Add(x=w547, y=200) -> (x+y=w545:i32)
          }
        }
        "intermediate residues" <- w503
        "Intermediate Best Fit" <- w505
        n188 = Bundle By Name(cluster=w511, "termination.max iteration"=w495, "termination.tolerance"=w494, "intermediate fits"=w500, "Intermediate Best Fit"=w505, "intermediate residues"=w503, "Intermediate delta"=w483) -> (w514:T5)
        n189 = call <vilib>:"Add State(s) to Queue__JKI_lib_State_Machine.vi"("State(s) in Front (\"\")"=w475, "State(s) in (\"\")"=w517) -> ("States Out"=w516:string)  [unwired: 13 in]
      }
      frame "Analysis: Iterate" {
        # "Iterate curve # and fit iteration #\nincrement fit iteration\nif fit iteration = 3, set to 0 and increment curve #\nif curve # is greater than the total # of curves end fitting"
        n190 = Unbundle By Name(w590) -> ("curve #"=w585:i32, "All G"=w584:cluster{dbl[], dbl[]}[], "fit iteration"=w588:i32, "Best Fit Parameters"=w579:dbl[][], "Intermediate Best Fit"=w581:dbl[][], "intermediate residues"=w580:dbl[], "residues"=w573:dbl[], "Intermediate delta"=w559:dbl[][], "delta best fit"=w556:dbl[][], "fits"=w560:cluster{dbl[], dbl[]}[], "intermediate fits"=w575:cluster{dbl[], dbl[]}[], "Initial curve?"=w571:bool, "Initial Best Fit"=w569:dbl[], "All locations"=w567:dbl[][], "Locations"=w568:dbl[], "Fit steps"=w564:i32[], "model step #"=w563:i32)
        n191 = Increment(x=w588) -> (x+1=w587:i32)
        n192 = case shown="4" w587 {
          selector: w587 -> [w608 _]
          tunnel: [w608 0] -> w586
          tunnel: w585 -> [w607 w624]
          tunnel: w584 -> [_ w651]
          tunnel: [w607 w647] -> w583
          tunnel: ["Analysis: Load data" w646] -> w554
          tunnel: w581 -> [w603 w622]
          tunnel: w580 -> [w605 w645]
          tunnel: w579 -> [w604 w644]
          tunnel: [w604 w643] -> w576
          tunnel: [w603 w612] -> w578
          tunnel: [w605 dbl[] [] ("residues")] -> w577
          tunnel: w560 -> [w602 w640]
          tunnel: w575 -> [w601 w641]
          tunnel: [w602 w638] -> w574
          tunnel: [w601 cluster{dbl[], dbl[]}[] [] ("intermediate fits")] -> w558
          tunnel: w573 -> [w600 w636]
          tunnel: [w600 w634] -> w572
          tunnel: w571 -> [w599 w632]
          tunnel: [w599 FALSE] -> w570
          tunnel: [w598 w631] -> w562
          tunnel: w569 -> [w598 w630]
          tunnel: w568 -> [_ w627]
          tunnel: w567 -> [w597 w628]
          tunnel: [w597 w626] -> w566
          tunnel: w564 -> [w596 w625]
          tunnel: [w596 w623] -> w565
          tunnel: w563 -> [_ _]
          tunnel: w559 -> [w595 w615]
          tunnel: [w595 w612] -> w557
          tunnel: w556 -> [w594 w613]
          tunnel: [w594 w611] -> w555
          frame 0, Default {
          }
          frame 4 {
            w612 = dbl[][] [] ("Intermediate Best Fit")
            n193 = Increment(x=w624) -> (x+1=w648:i32)
            n194 = Array Size(array=w651) -> (size(s)=w649:i32)
            n195 = Array Max & Min(array=w645) -> (min value=w635:dbl, min index (indices)=w614:i32)  [unwired: 2 out]
            n196 = Less?(x=w648, y=w649) -> (x < y?=w650:bool)
            n197 = Index Array(array=w641, index=w614) -> (element=w639:cluster{dbl[], dbl[]})
            n198 = Index Array(array=w622, index (row)=w614) -> (element=w618:dbl[])  [unwired: 1 in]
            n199 = Index Array(array=w615, index (row)=w614) -> (element=w610:dbl[])  [unwired: 1 in]
            n200 = case shown="True" w632 {
              tunnel: w618 -> [w654 w657]
              tunnel: [w655 w657] -> w631
              tunnel: w630 -> [w655 _]
              tunnel: [w654 w656] -> w629
              tunnel: w610 -> [w653 _]
              tunnel: [w653 w656] -> w609
              frame False {
              }
              frame True {
                w656 = dbl[] [] ("residues")
              }
            }
            n201 = case shown="True" w650 {
              tunnel: w648 -> [_ w660]
              tunnel: [0 w660] -> w647
              tunnel: ["Display: Fit" "Analysis: Load data"] -> w646
              frame False {
              }
              frame True {
              }
            }
            n202 = call-poly <userlib>:"Filter 1D Array__ogtk.vi"("items to filter"=0, "array"=w618) -> ("filtered array"=w617:dbl[])  [unwired: 4 in, 1 out]
            n203 = Build Array (concatenate)(w628, w627) -> (w626:dbl[][])
            n204 = Build Array (concatenate)(w636, w635) -> (w634:dbl[])
            n205 = Array Size(array=w617) -> (size(s)=w621:i32)
            n206 = Build Array (concatenate)(w640, w639) -> (w638:cluster{dbl[], dbl[]}[])
            n207 = Build Array (concatenate)(w613, w609) -> (w611:dbl[][])
            n208 = Divide(x=w621, y=3) -> (x/y=w619:dbl)
            n209 = Build Array (concatenate)(w644, w629) -> (w643:dbl[][])
            n210 = Build Array (concatenate)(w625, w619) -> (w623:dbl[])
          }
        }
        "Best Fit Parameters" <- w576
        "residues" <- w572
        "Initial Best Fit" <- w562
        "Fit steps" <- w565
        "delta best fit" <- w555
        n211 = call <vilib>:"Add State(s) to Queue__JKI_lib_State_Machine.vi"("State(s) in Front (\"\")"=w554, "State(s) in (\"\")"=w593) -> ("States Out"=w592:string)  [unwired: 13 in]
        n212 = local write "fits"(w574) -> ()
        n213 = call "parse best fit into string array.vi"("Initial Best Fit"=w562) -> ("concatenated string"=→"initial best fit":string)  [unwired: 10 in]
        n214 = Bundle By Name(cluster=w590, "curve #"=w583, "fit iteration"=w586, "termination"=cluster{"max iteration":i32, "tolerance":dbl} {"max iteration"=200, "tolerance"=1e-08}, "Best Fit Parameters"=w576, "Intermediate Best Fit"=w578, "intermediate residues"=w577, "residues"=w572, "Intermediate delta"=w557, "delta best fit"=w555, "intermediate fits"=w558, "fits"=w574, "Initial curve?"=w570, "Initial Best Fit"=w562, "All locations"=w566, "Fit steps"=w565) -> (w591:T5)
      }
      frame "----------Display-------------" {
        # "Your code here.\n(You can make a copy of, or modify, this frame)"
        n215 = call <vilib>:"Add State(s) to Queue__JKI_lib_State_Machine.vi"("State(s) in (\"\")"=w665) -> ("States Out"=w664:string)  [unwired: 14 in]
      }
      frame "Display: Fit" {
        # "place holder for B field values"
        # "extract and sort Vsg peak values"
        n216 = Unbundle By Name(w723) -> ("All G"=w721:cluster{dbl[], dbl[]}[], "fits"=w716:cluster{dbl[], dbl[]}[], "Best Fit Parameters"=w714:dbl[][], "residues"=w713:dbl[], "one width?"=w670:bool, "delta best fit"=w669:dbl[][])  [unwired: 1 out]
        n217 = Index Array(array=w713, index="display index") -> (element=→"Display residue":dbl)
        n218 = Array Size(array=w713) -> (size(s)=w712:i32)
        n219 = for {
          N: w712 -> [_]
          tunnel: [w804] -> w667 mode=indexing
          i -> [w806]
          n220 = local read "B multiplier"() -> (w802:dbl)
          n221 = local read "B offset"() -> (w803:dbl)
          n222 = Multiply(x=w802, y=w806) -> (x*y=w805:dbl)
          n223 = Add(x=w803, y=w805) -> (x+y=w804:dbl)
        }
        n224 = case shown="False" w670 {
          tunnel: [w733 w765] -> w715
          tunnel: w714 -> [w732 w764]
          tunnel: w712 -> [w731 w763]
          tunnel: [w730 w762] -> w681
          tunnel: [w729 w761] -> w679
          tunnel: w669 -> [w728 w760]
          tunnel: [w727 w759] -> w668
          frame False {
            n225 = for {
              N: w731 -> [_]
              tunnel: w732 -> [w758]
              tunnel: [w751] -> w733 mode=indexing
              tunnel: [w748] -> w730 mode=indexing
              tunnel: [w746] -> w729 mode=indexing
              tunnel: w728 -> [w745]
              tunnel: [w734] -> w727 mode=indexing
              i -> [w744]
              w742 = 0.0
              w753 = 0.0
              n226 = Index Array(array=w758, index (row)=w744) -> (element=w757:dbl[])  [unwired: 1 in]
              n227 = Index Array(array=w745, index (row)=w744) -> (element=w743:dbl[])  [unwired: 1 in]
              n228 = Decimate 1D Array(w757) -> (w755:dbl[], w756:dbl[], w754:dbl[])
              n229 = Decimate 1D Array(w743) -> (w741:dbl[], w740:dbl[], w739:dbl[])
              n230 = call-poly <userlib>:"Filter 1D Array__ogtk.vi"("items to filter"=w742, "array"=w739) -> ("filtered array"=w737:dbl[])  [unwired: 4 in, 1 out]
              n231 = call-poly <userlib>:"Filter 1D Array__ogtk.vi"("items to filter"=w753, "array"=w754) -> ("filtered array"=w747:dbl[])  [unwired: 4 in, 1 out]
              n232 = call-poly <userlib>:"Filter 1D Array__ogtk.vi"("items to filter"=w742, "array"=w741) -> ("filtered array"=w735:dbl[])  [unwired: 4 in, 1 out]
              n233 = call-poly <userlib>:"Filter 1D Array__ogtk.vi"("items to filter"=w742, "array"=w740) -> ("filtered array"=w736:dbl[])  [unwired: 4 in, 1 out]
              n234 = call-poly <userlib>:"Filter 1D Array__ogtk.vi"("items to filter"=w753, "array"=w756) -> ("filtered array"=w752:dbl[])  [unwired: 4 in, 1 out]
              n235 = call-poly <userlib>:"Filter 1D Array__ogtk.vi"("items to filter"=w753, "array"=w755) -> ("filtered array"=w749:dbl[])  [unwired: 4 in, 1 out]
              n236 = call-poly <userlib>:"Sort Array__ogtk.vi"("Order"=enum16{"ascending", "descending"}."ascending", "Array in"=w752) -> ("Sorted Pointers"=w738:i32[], "Sorted Array out"=w751:dbl[])  [unwired: 8 in]
              n237 = call-poly <userlib>:"Reorder Array2__ogtk.vi"("indices"=w738, "array"=w735) -> ()  [unwired: 9 in, 1 out]
              n238 = call-poly <userlib>:"Reorder Array2__ogtk.vi"("indices"=w738, "array"=w736) -> ("reordered array"=w734:dbl[])  [unwired: 9 in]
              n239 = call-poly <userlib>:"Reorder Array2__ogtk.vi"("indices"=w738, "array"=w737) -> ()  [unwired: 9 in, 1 out]
              n240 = call-poly <userlib>:"Reorder Array2__ogtk.vi"("indices"=w738, "array"=w747) -> ("reordered array"=w746:dbl[])  [unwired: 9 in]
              n241 = call-poly <userlib>:"Reorder Array2__ogtk.vi"("indices"=w738, "array"=w749) -> ("reordered array"=w748:dbl[])  [unwired: 9 in]
            }
          }
          frame True {
            n242 = for {
              N: w763 -> [_]
              tunnel: w764 -> [w792]
              tunnel: [w775] -> w765 mode=indexing
              tunnel: [w774] -> w762 mode=indexing
              tunnel: [w784] -> w761 mode=indexing
              tunnel: w760 -> [w783]
              tunnel: [w766] -> w759 mode=indexing
              i -> [w782]
              w770 = 0.0
              w789 = 0.0
              n243 = Index Array(array=w783, index (row)=w782) -> (element=w781:dbl[])  [unwired: 1 in]
              n244 = Index Array(array=w792, index (row)=w782) -> (element=w788:dbl[])  [unwired: 1 in]
              n245 = Delete From Array(array=w788, length=1, index=0) -> (deleted portion=w784:dbl[], array with subset deleted=w785:dbl[])
              n246 = Delete From Array(array=w781, length=1, index=0) -> (array with subset deleted=w778:dbl[])  [unwired: 1 out]
              n247 = Decimate 1D Array(w785) -> (w790:dbl[], w791:dbl[])
              n248 = Decimate 1D Array(w778) -> (w772:dbl[], w771:dbl[])
              n249 = call-poly <userlib>:"Filter 1D Array__ogtk.vi"("items to filter"=w789, "array"=w791) -> ("filtered array"=w777:dbl[])  [unwired: 4 in, 1 out]
              n250 = call-poly <userlib>:"Filter 1D Array__ogtk.vi"("items to filter"=w789, "array"=w790) -> ("filtered array"=w776:dbl[])  [unwired: 4 in, 1 out]
              n251 = call-poly <userlib>:"Filter 1D Array__ogtk.vi"("items to filter"=w770, "array"=w772) -> ("filtered array"=w769:dbl[])  [unwired: 4 in, 1 out]
              n252 = call-poly <userlib>:"Filter 1D Array__ogtk.vi"("items to filter"=w770, "array"=w771) -> ("filtered array"=w768:dbl[])  [unwired: 4 in, 1 out]
              n253 = call-poly <userlib>:"Sort Array__ogtk.vi"("Order"=enum16{"ascending", "descending"}."ascending", "Array in"=w777) -> ("Sorted Pointers"=w767:i32[], "Sorted Array out"=w775:dbl[])  [unwired: 8 in]
